vi "FITS - Define FITS Keywords.vi"() -> (0 "Extension Comments":string[](array[string])=["", "BITS PER PIXEL", "NUMBER OF AXES (2)", "XDIM (PIXELS)", "YDIM (PIXELS)", "4 POLARIZATION STATES", "", "TIME OF OBSERVATION (UTC)", "DATE OF OBSERVATION END (UTC)", "EXPOSURE TIME (MILLISEC)", "", "32768.", "1", "NUMBER OF IMAGES AT EACH STATE", "WAVELENGTH OF OBS (NM)", "", "", "", "", "", "", "", "", "", "", "", "", "", ""], 1 "Extension  Keywords":string[](array[string])=["XTENSION", "BITPIX", "NAXIS", "NAXIS1", "NAXIS2", "NAXIS3", "GCOUNT", "TIME_OBS", "DATE_END", "EXPOSURE", "PCOUNT", "BZERO", "BSCALE", "MODC", "WAVELENG", "COMMENT", "COMMENT", "COMMENT", "COMMENT", "COMMENT", "COMMENT", "COMMENT", "COMMENT", "COMMENT", "COMMENT", "COMMENT", "COMMENT", "COMMENT", "COMMENT"], 2 "Primary Comments":string[](array[string])=["CONFORMS TO FITS STANDARD", "BITS PER PIXEL", "DATA DIMENSIONS IN FITS FILE", "XDIM (PIXELS)", "YDIM (PIXELS)", "4 POLARIZATION STATES", "1 CAMERA", "EXTENSIONS POSSIBLE", "NAME OF OBSERVER", "NAME OF TELESCOPE", "LOCATION OF TELESCOPE", "NAME OF INSTRUMENT", " ADU OFFSET", "CAMERA-STAGE POSITION (MM)", "ROTATIONAL POSITION (DEG)", "0=IN BEAM, 1=OUT OF BEAM", "PRE-FILTER CENTER WAVELENGTH (NM)", "CAL-WHEEL POSITION", "CAMERA SERIAL NUMBER", "FOCAL PLANE TEMP (C)", "LCVR RELAXATION DELAY (mS)", "DATE OF OBSERVATION START (UTC)", "TIME OF OBSERVATION (UTC)", "EXPOSURE TIME (S)", "NUMBER OF IMAGES AT EACH STATE", "TUNING VOLTAGE-1", "TUNING VOLTAGE-2", "TUNING VOLTAGE-3", "TUNING VOLTAGE-4", "TUNING VOLTAGE-5", "BEAM (0=ON BAND OR 1=CONTINUUM)", "WAVELENGTH OF OBS (NM)", "OBSERVER COMMENT", "COOKBOOK  LOADED", "IMAGE TYPE", "SCIENTIFIC GROUP"], 3 "Primary Keywords":string[](array[string])=["SIMPLE", "BITPIX", "NAXIS", "NAXIS1", "NAXIS2", "NAXIS3", "NAXIS4", "EXTEND", "OBSERVER", "TELESCOP", "LOCATION", "INSTRUME", "BZERO", "FOCUS", "ROTPOS", "DIFFUSER", "FW-WVLNG", "FW-CALIB", "CAM-SN1", "CAM-TEMP", "TUNEDLAY", "DATE_OBS", "TIME_OBS", "EXPOSURE", "MODC", "NLC-1", "NLC-2", "NLC-3", "NLC-4", "NLC-5", "BEAM", "WAVELENG", "COMMHEAD", "COOKBOOK", "DATATYPE", "ORIGIN"], 4 "Number of Extension keywords":i32=29, 5 "Number of Primary keywords":i32=36)   [LabVIEW 2014]
panel:
  in  "Extension Header":string[][](table)=[["XTENSION", ""], ["BITPIX", "BITS PER PIXEL"], ["NAXIS", "NUMBER OF AXES (2)"], ["NAXIS1", "XDIM (PIXELS)"], ["NAXIS2", "YDIM (PIXELS)"], ["NAXIS3", "4 POLARIZATION STATES"], ["GCOUNT", ""], ["TIME_OBS", "TIME OF OBSERVATION (UTC)"], ["DATE_END", "DATE OF OBSERVATION END (UTC)"], ["EXPOSURE", "EXPOSURE TIME (S)"], ["PCOUNT", ""], ["", ""], ["BZERO", "32768."], ["BSCALE", "1"], ["MODC", "NUMBER OF IMAGES AT EACH STATE"], ["WAVELENG", "WAVELENGTH OF OBS (NM)"], ["", ""], ["", ""], ["", ""], ["", ""], ["", ""], ["COMMENT", ""], ["COMMENT", ""], ["COMMENT", ""], ["COMMENT", ""], ["COMMENT", ""], ["COMMENT", ""], ["COMMENT", ""], ["COMMENT", ""], ["COMMENT", ""], ["COMMENT", ""], ["COMMENT", ""], ["COMMENT", ""], ["COMMENT", ""], ["COMMENT", ""], ["", ""], ["", ""]]
  in  "Primary Header":string[][](table)=[["SIMPLE", "CONFORMS TO FITS STANDARD"], ["BITPIX", "BITS PER PIXEL"], ["NAXIS", "DATA DIMENSIONS IN FITS FILE"], ["NAXIS1", "XDIM (PIXELS)"], ["NAXIS2", "YDIM (PIXELS)"], ["NAXIS3", "4 POLARIZATION STATES"], ["NAXIS4", "1 CAMERA"], ["EXTEND", "EXTENSIONS POSSIBLE"], ["OBSERVER", "NAME OF OBSERVER"], ["TELESCOP", "NAME OF TELESCOPE"], ["LOCATION", "LOCATION OF TELESCOPE"], ["INSTRUME", "NAME OF INSTRUMENT"], ["BZERO", " ADU OFFSET"], ["FOCUS", "CAMERA-STAGE POSITION (MM)"], ["ROTPOS", "ROTATIONAL POSITION (DEG)"], ["DIFFUSER", "0=IN BEAM, 1=OUT OF BEAM"], ["FW-WVLNG", "PRE-FILTER CENTER WAVELENGTH (NM)"], ["FW-CALIB", "CAL-WHEEL POSITION"], ["CAM-SN1", "CAMERA SERIAL NUMBER"], ["CAM-TEMP", "FOCAL PLANE TEMP (C)"], ["TUNEDLAY", "LCVR RELAXATION DELAY (mS)"], ["DATE_OBS", "DATE OF OBSERVATION START (UTC)"], ["TIME_OBS", "TIME OF OBSERVATION (UTC)"], ["EXPOSURE", "EXPOSURE TIME (S)"], ["MODC", "NUMBER OF IMAGES AT EACH STATE"], ["NLC-1", "TUNING VOLTAGE-1"], ["NLC-2", "TUNING VOLTAGE-2"], ["NLC-3", "TUNING VOLTAGE-3"], ["NLC-4", "TUNING VOLTAGE-4"], ["NLC-5", "TUNING VOLTAGE-5"], ["BEAM", "BEAM (0=ON BAND OR 1=CONTINUUM)"], ["WAVELENG", "WAVELENGTH OF OBS (NM)"], ["COMMHEAD", "OBSERVER COMMENT"], ["COOKBOOK", "COOKBOOK  LOADED"], ["DATATYPE", "IMAGE TYPE"], ["ORIGIN", "SCIENTIFIC GROUP"]]
  # "Primay Keywords are used for those instrumental descriptors which change only very\nslowly or not at all during an experiment."
  # "Extension Keywords are used for those observational parameters which change on the order\nof the modulation frequency (20 Hz)"
  # "36 Keywords will give a header that is a\nmultiple of 2880 if each keyword is 80 characters"
  # "(does not include END)"
  # "(does not include END)"
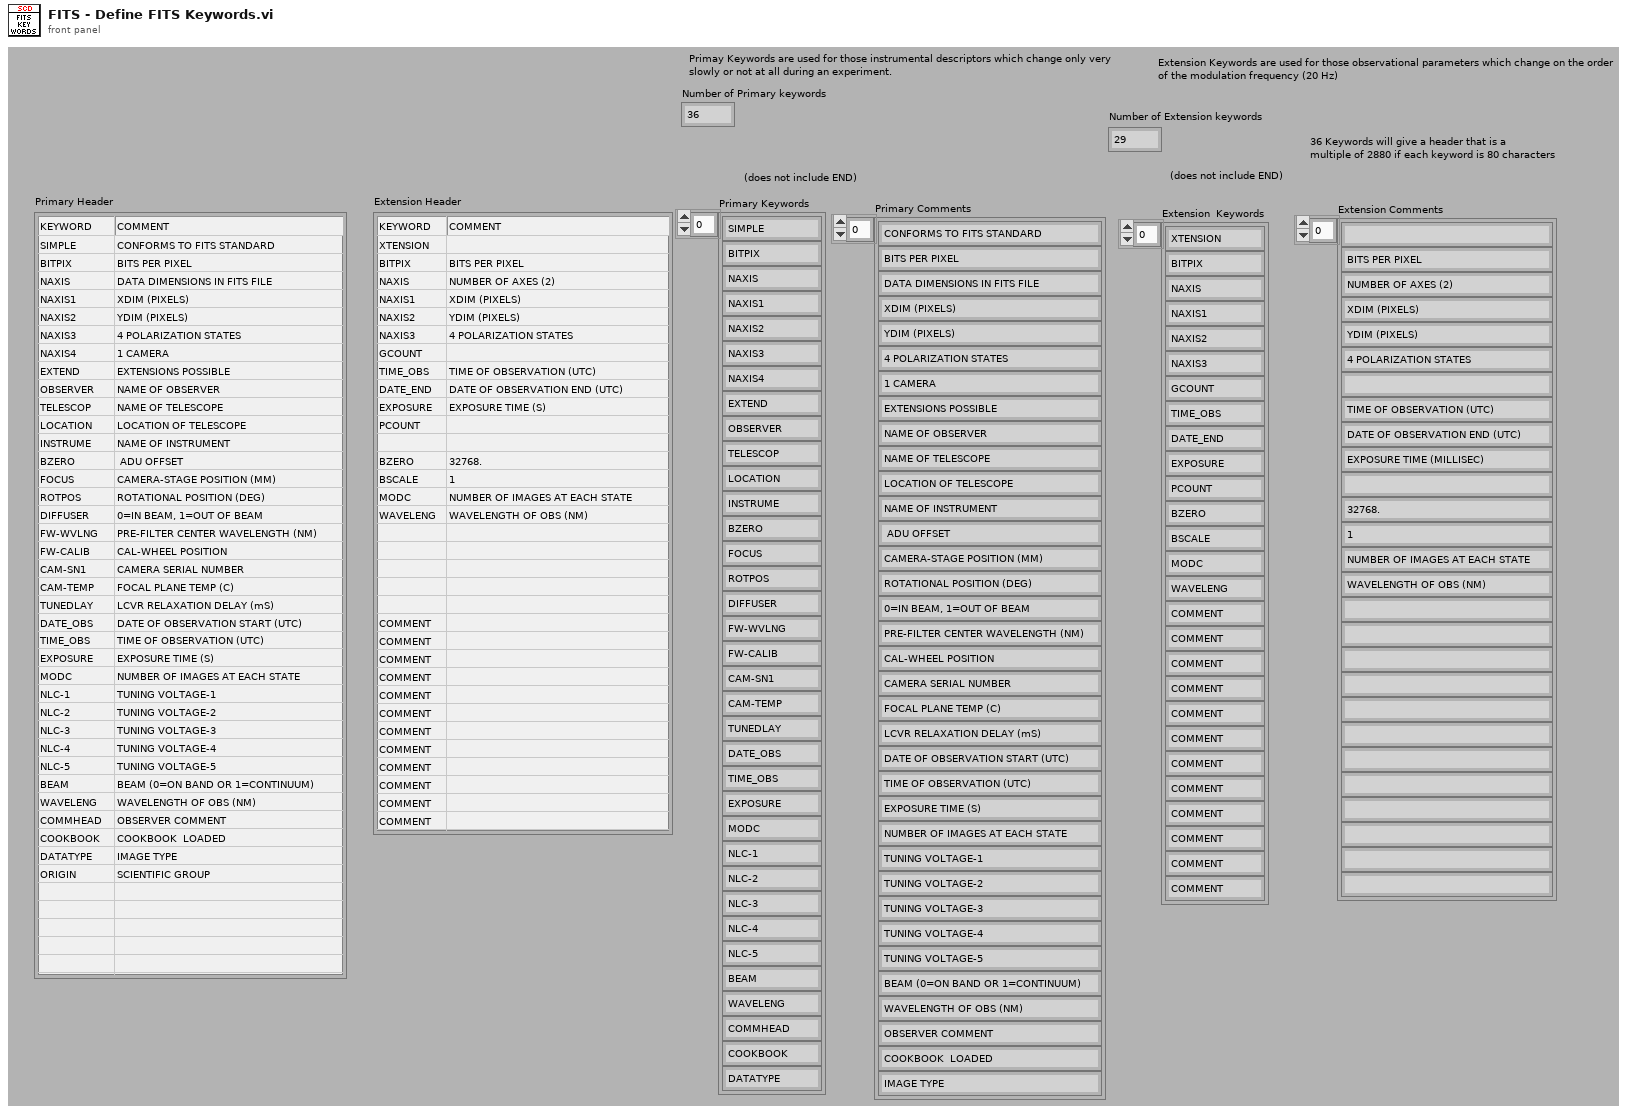
[diagram p1: front panel]
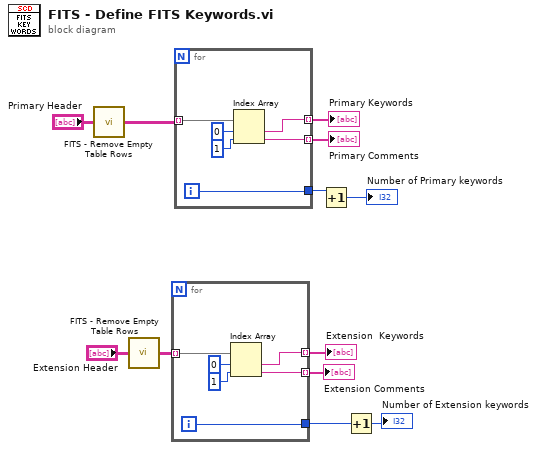
[diagram p0: block diagram]
diagram:
  n1 = call "FITS - Remove Empty Table Rows.vi"("Table"="Primary Header") -> ("Table with empty trailers removed"=w11:string[][])
  n2 = call "FITS - Remove Empty Table Rows.vi"("Table"="Extension Header") -> ("Table with empty trailers removed"=w6:string[][])
  n3 = for {
    tunnel: w6 -> [w18] mode=indexing
    tunnel: [w15] -> w5 mode=indexing
    tunnel: [w14] -> w4 mode=indexing
    tunnel: [w13] -> w3
    i -> [w13]
    n4 = Index Array(array=w18, index #1=0 ("index"), index #2=1 ("index")) -> (element #1=w15:string, element #2=w14:string)
  }
  "Extension Comments" <- w4
  "Extension  Keywords" <- w5
  n5 = for {
    tunnel: w11 -> [w24] mode=indexing
    tunnel: [w21] -> w8 mode=indexing
    tunnel: [w20] -> w10 mode=indexing
    tunnel: [w19] -> w9
    i -> [w19]
    n6 = Index Array(array=w24, index #1=0 ("index"), index #2=1 ("index")) -> (element #1=w21:string, element #2=w20:string)
  }
  "Primary Keywords" <- w8
  "Primary Comments" <- w10
  n7 = Increment(x=w9) -> (x+1=→"Number of Primary keywords":i32)
  n8 = Increment(x=w3) -> (x+1=→"Number of Extension keywords":i32)
